vi "UtilityLib.GUI styles and colors example.vi"() -> ()   [LabVIEW 2014, in "UtilityLib.lvlib"]
doc: "This routine demonstrates usage of colors and gives some guidelines for GUIs. Moreover it demonstrates the usage of \"set colors of panel to defaults\""
uses:
  UtilityLib.lvlib
  UtilityLib.valueStatus.ctl
panel:
  out "aModernString":string
  out "aClassicString":string
  out "aString":string="warning"
  out "stringArrayModern":string[](array[string])=["a", "b", "c"]
  out "numericArrayModern":dbl[](array[numeric])=[1.0, 2.0, 3.0]
  out "stringArrayClassic":string[](array[string])=["a", "b", "c"]
  out "numericArrayClassic":dbl[](array[numeric])=[1.0, 2.0, 3.0]
  in  "Numeric 8":dbl
  in  "Numeric 7":dbl
  in  "Numeric 6":dbl
  in  "Numeric 5":dbl
  in  "Numeric 4":dbl
  in  "Numeric 3":dbl
  in  "Numeric 2":dbl
  in  "Numeric":dbl
  in  "Stop":bool
  out "indicator":string="another string"
  in  "control":string="a string"
  out "aSimpleStringFromClassicP":string="warning"
  in  "valueStatus":T1=enum."indicator default"
  out "Multicolumn Listbox":i32(listbox)=-1
  # "1) use SYSTEM color as background color"
  # "2) Listbox: use CLASSIC listboxes and tables. See diagram for coloring."
  # "Please note the following:\n- The colors\n-- red (error/alarm/malfunction), and\n-- yellow (warning) are really reserved. \n    !! Don't use red and yellow for something else !!\n\n- The color pink (important information) is rather ugly. However,\n  it is the only color that is unique and not used for something else.\n\n- blinking of indicators, controls, etc. is STRICTLY RESERVED  for warnings \n  (slow blinking) and errors (fast blinking).\n  !! Blinking is the only means to inform color blind people of an error or warning !!"
  # "3) Control buttons: use MODERN buttons with 3DObject colors (which is anyhow LabVIEW default)"
  # "4) Use \"simple\" string and numeric indicators from the CLASSIC palette. They need little space and don't have space consuming frames"
  # "4.1) You may use coloring for indicators"
  # "4.2) DON'T USE TOO MANY COLORS! Typically,  controls and indicators look like this (which is anyhow LabVIEW default)"
  # "4.3) Consider using elements from the CLASSIC palette, since they need less space. However, use consistent style within one GUI."
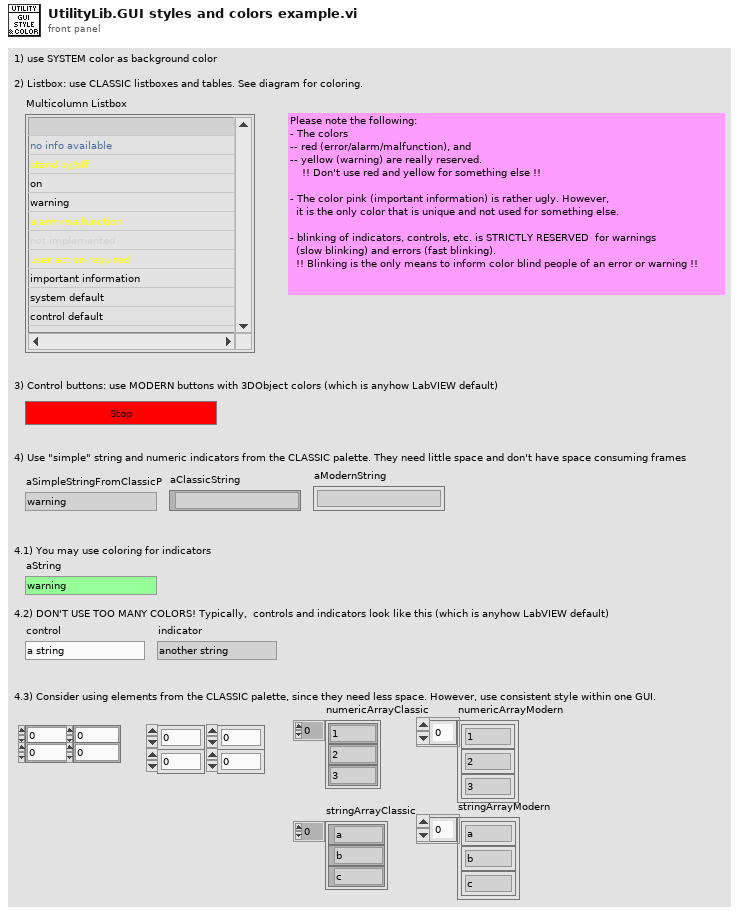
[diagram p1: front panel]
types:
  T1 = typedef "UtilityLib.lvlib/UtilityLib.valueStatus.ctl" = enum16{"no info available", "stand by/off", "on", "warning", "alarm/malfunction", "not implemented", "user action required", "important information", "system default", "control default", "indicator default", "button default"}
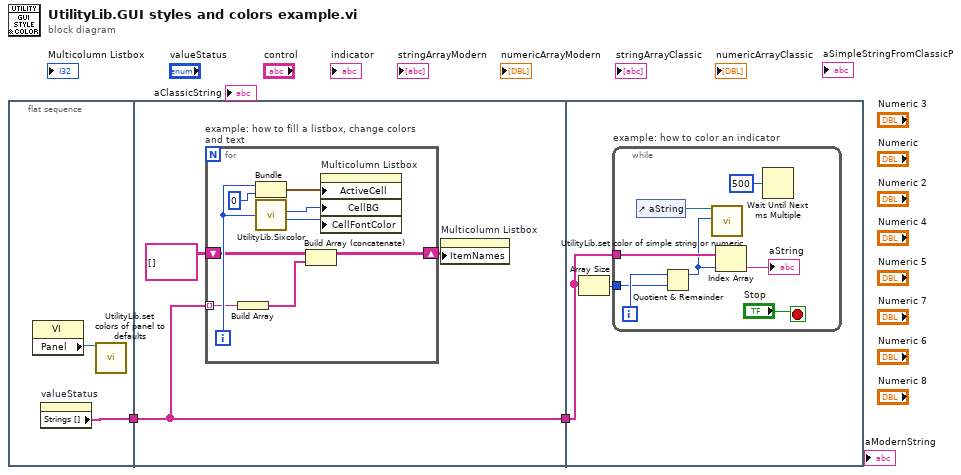
[diagram p0: block diagram]
diagram:
  n1 = flat-sequence {
    tunnel: [w3] -> w2
    tunnel: w2 -> [w5]
    tunnel: [w5] -> w1
    tunnel: w1 -> [w17]
    frame #0 {
      n2 = property class="VI"() -> ("Panel"=w4:refnum<vi>)  [unwired: 2 in, 2 out]
      n3 = property on="valueStatus" class="Enum (strict)"() -> ("Strings []"=w3:string[])  [unwired: 2 in, 2 out]
      n4 = call "UtilityLib.set colors of panel to defaults.vi"("Front Panel"=w4) -> ()  [unwired: 18 in, 1 out]
    }
    frame #1 {
      n5 = for "example: how to fill a listbox, change colors and text" {
        tunnel: w5 -> [w9] mode=indexing
        shift-right: [w10] -> w6
        shift-left: string[][] [] ("Item Names") -> [w11]
        i -> [w12]
        n6 = Build Array(w9) -> (w8:string[])
        n7 = Bundle(w12, 0) -> (w16:cluster{i32, i32})  [unwired: 1 in]
        n8 = call "UtilityLib.Sixcolor.vi"("State"=w12) -> ("elementBackground"=w14:u32, "elementText"=w13:u32)  [unwired: 2 in, 2 out]
        n9 = Build Array (concatenate)(w11, w8) -> (w10:string[][])
        n10 = property on="Multicolumn Listbox" class="MCListbox (strict)"("ActiveCell"=w16, "CellBG"=w14, "CellFontColor"=w13) -> ()  [unwired: 2 in, 2 out]
      }
      n11 = property on="Multicolumn Listbox" class="MCListbox (strict)"("ItemNames"=w6) -> ()  [unwired: 2 in, 2 out]
    }
    frame #2 {
      n12 = Array Size(array=w17) -> (size(s)=w18:i32)
      n13 = while "example: how to color an indicator" {
        tunnel: w18 -> [w25]
        tunnel: w17 -> [w23]
        i -> [w26]
        stop <- "Stop" stop-if-true
        n14 = control-ref of="aString"() -> (w24:refnum<vi>)
        n15 = Quotient & Remainder(x=w26, y=w25) -> (x-y*floor(x/y)=w22:i32)  [unwired: 1 out]
        n16 = call "UtilityLib.set color of simple string or numeric.vi"("simpleString"=w24, "valueStatus"=w22) -> ()  [unwired: 17 in, 1 out]
        n17 = Index Array(array=w23, index=w22) -> (element=→"aString":string)
        n18 = Wait Until Next ms Multiple(millisecond multiple=u32 500) -> ()  [unwired: 1 out]
      }
    }
  }
